vi "Update Intensity Plot.vi"(9 "Z":dbl[](array[numeric]), 10 "FEM Grid":T1, 11 "FEM plot in":refnum<vi>) -> (3 "FEM plot out":refnum<vi>)   [LabVIEW 2020, in "Heat Equation Solver.lvlib"]
uses:
  Heat Equation Solver.lvlib
  FEM Grid.ctl
  <vilib>/Analysis/baseanly.llb/Mean (DBL).vi
  <vilib>/picture/3D Picture Control/Object/Create Object (name).vi
  <vilib>/picture/3D Picture Control/NI_3D Picture Control.lvlib
  <vilib>/Analysis/NI_AALBase.lvlib
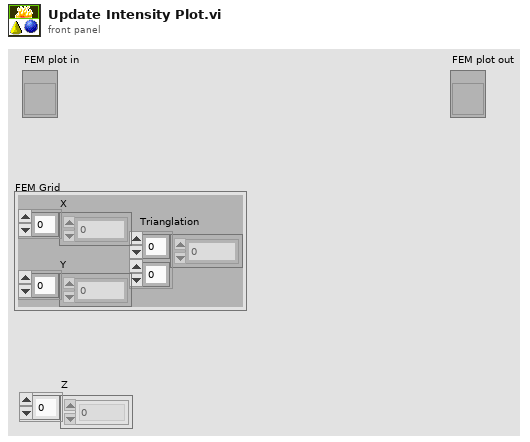
[diagram p1: front panel]
types:
  T1 = typedef "Heat Equation Solver.lvlib/FEM Grid.ctl" = cluster{"X":dbl[], "Y":dbl[], "Trianglation":i32[][]}
  T2 = enum16{"Inherit Value", "Points", "Wireframe", "Polygons"}
  T3 = enum16{"Overall", "Per Primitive", "Per Vertex", "Binding Off"}
  T4 = enum16{"Points", "Lines", "Line Strip", "Line Loop", "Triangles", "Triangle Strip", "Triangle Fan", "Quads", "Quad Strip", "Polygon"}
  T5 = cluster{"Numeric":dbl, "Numeric":dbl, "Numeric":dbl}
  T6 = typedef "LVRGBAColorTypeDef.ctl" = cluster{"Red":sgl, "Green":sgl, "Blue":sgl, "Alpha":sgl}
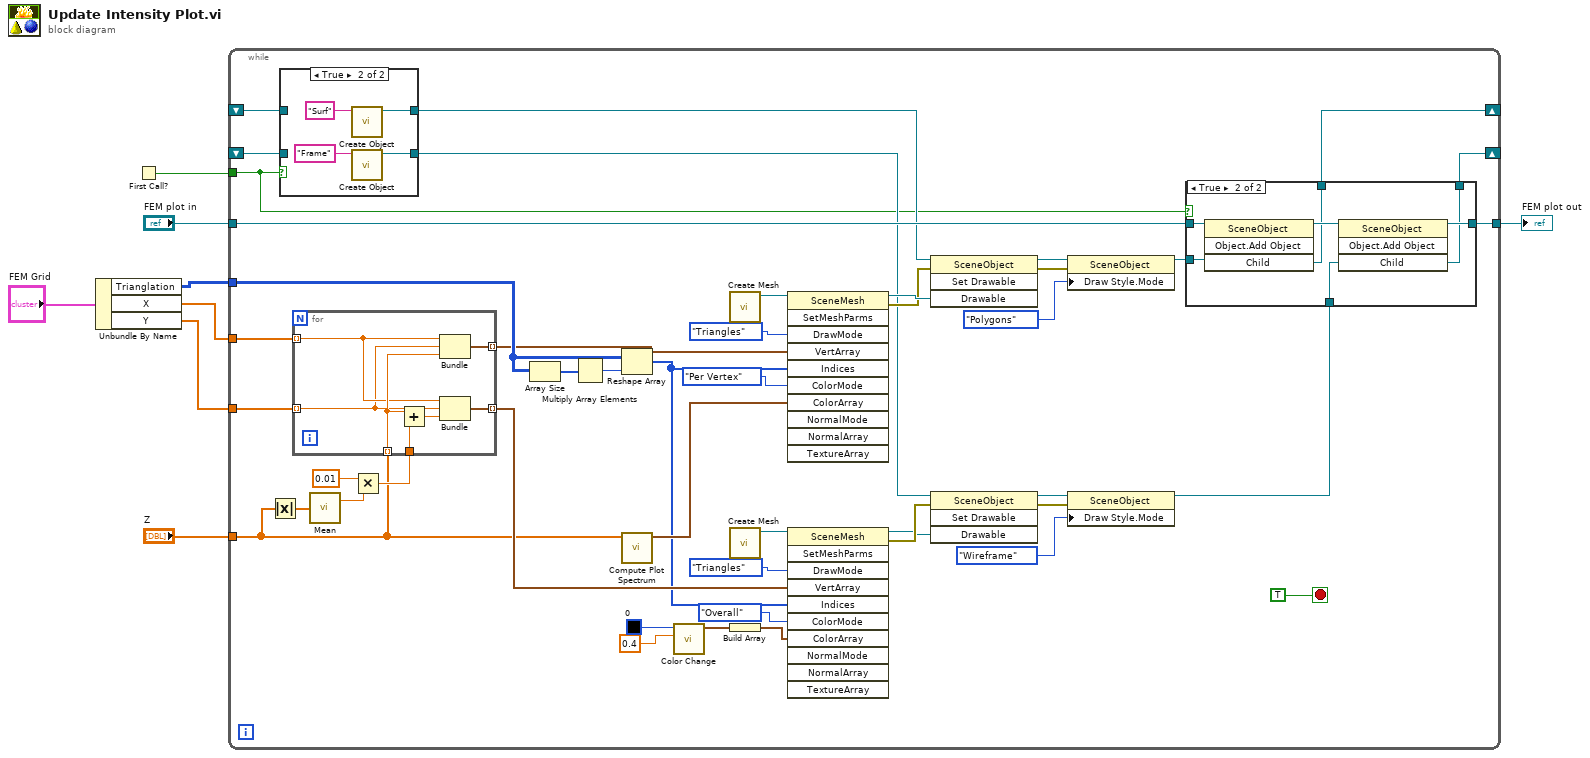
[diagram p0: block diagram]
diagram:
  n1 = Unbundle By Name("FEM Grid") -> ("Trianglation"=w3:i32[][], "X"=w2:dbl[], "Y"=w1:dbl[])
  n2 = First Call?() -> (First Call?: T/F=w5:bool)
  n3 = while {
    tunnel: w3 -> [w44]
    tunnel: "FEM plot in" -> [w25]
    tunnel: [w24] -> w7
    tunnel: "Z" -> [w19]
    tunnel: w2 -> [w18]
    tunnel: w1 -> [w17]
    tunnel: w5 -> [w11]
    shift-right: [w15] -> _
    shift-left: _ -> [w14]
    shift-right: [w12] -> _
    shift-left: _ -> [w10]
    stop <- TRUE stop-if-true
    n4 = Absolute Value(x=w19) -> (abs(x)=w20:dbl[])
    n5 = case shown="True" w11 {
      tunnel: [w66 w70] -> w16
      tunnel: w14 -> [w66 _]
      tunnel: [w65 w69] -> w13
      tunnel: w10 -> [w65 _]
      frame False {
      }
      frame True {
        n6 = call-poly <vilib>:"Create Object.vi"("Name"="Surf") -> ("Scene:New Object"=w70:refnum<vi>)  [unwired: 9 in, 1 out]
        n7 = call-poly <vilib>:"Create Object.vi"("Name"="Frame") -> ("Scene:New Object"=w69:refnum<vi>)  [unwired: 9 in, 1 out]
      }
    }
    n8 = call-poly <vilib>:"Mean.vi"("X"=w20) -> ("mean"=w23:dbl)  [unwired: 1 out]
    n9 = Multiply(x=0.01 ("y"), y=w23) -> (x*y=w21:dbl)
    n10 = for {
      tunnel: w19 -> [w76] mode=indexing
      tunnel: [w77] -> w34 mode=indexing
      tunnel: [w74] -> w33 mode=indexing
      tunnel: w21 -> [w73]
      tunnel: w18 -> [w72] mode=indexing
      tunnel: w17 -> [w71] mode=indexing
      n11 = Add(x=w76, y=w73) -> (x+y=w75:dbl)
      n12 = Bundle("Numeric"=w72, "Numeric"=w71, "Numeric"=w76) -> (w77:T5)  [unwired: 1 out]
      n13 = Bundle("Numeric"=w72, "Numeric"=w71, w75) -> (w74:cluster{"Numeric":dbl, "Numeric":dbl, dbl})  [unwired: 1 out]
    }
    n14 = Array Size(array=w44) -> (size(s)=w51:i32[])
    n15 = Multiply Array Elements(1:w51) -> (0:w50:i32)
    n16 = Reshape Array(w44, w50) -> (w32:i32[])
    n17 = call "Compute Plot Spectrum.vi"("U(x, y)"=w19) -> ("Color Array"=w45:T6[])  [unwired: 10 in]
    n18 = call <vilib>:"Color Change.vi"("Alpha"=0.4, "Color"=u32 0) -> ("RGBA"=w31:cluster{"R":sgl, "G":sgl, "B":sgl, "A":sgl})  [unwired: 9 in]
    n19 = call <vilib>:"Create Mesh.vi"() -> ("New Mesh Refnum"=w54:refnum<vi>)  [unwired: 1 in, 10 out]
    n20 = call <vilib>:"Create Mesh.vi"() -> ("New Mesh Refnum"=w35:refnum<vi>)  [unwired: 1 in, 10 out]
    n21 = Build Array(w31) -> (w30:cluster{"R":sgl, "G":sgl, "B":sgl, "A":sgl}[])
    n22 = invoke class="SceneMesh" method="SetMeshParms"(reference=w54, "DrawMode"=T4."Triangles" ("Draw Mode"), "VertArray"=w34, "Indices"=w32, "ColorMode"=T3."Per Vertex" ("Color Binding Mode"), "ColorArray"=w45) -> (reference out=w53:refnum<vi>, error out=w46:errorcluster)  [unwired: 5 in, 9 out]
    n23 = invoke class="SceneMesh" method="SetMeshParms"(reference=w35, "DrawMode"=T4."Triangles" ("Draw Mode"), "VertArray"=w33, "Indices"=w32, "ColorMode"=T3."Overall" ("Color Binding Mode"), "ColorArray"=w30) -> (reference out=w36:refnum<vi>, error out=w41:errorcluster)  [unwired: 5 in, 9 out]
    n24 = invoke class="SceneObject" method="Set Drawable"(reference=w16, error in=w46, "Drawable"=w53) -> (reference out=w52:refnum<vi>, error out=w47:errorcluster)  [unwired: 1 in, 2 out]
    n25 = invoke class="SceneObject" method="Set Drawable"(reference=w13, error in=w41, "Drawable"=w36) -> (reference out=w37:refnum<vi>, error out=w40:errorcluster)  [unwired: 1 in, 2 out]
    n26 = property class="SceneObject"(reference=w52, error in=w47, "Draw Style.Mode"=T2."Polygons" ("Draw Style:Mode")) -> (reference out=w27:refnum<vi>)  [unwired: 1 out]
    n27 = property class="SceneObject"(reference=w37, error in=w40, "Draw Style.Mode"=T2."Wireframe" ("Draw Style:Mode")) -> (reference out=w26:refnum<vi>)  [unwired: 1 out]
    n28 = case shown="True" w11 {
      tunnel: w27 -> [w57 w63]
      tunnel: w26 -> [w56 w62]
      tunnel: w25 -> [w55 w61]
      tunnel: [w55 w60] -> w24
      tunnel: [w57 w59] -> w15
      tunnel: [w56 w58] -> w12
      frame False {
      }
      frame True {
        n29 = invoke class="SceneObject" method="Object.Add Object"(reference=w61, "Child"=w63) -> (reference out=w64:refnum<vi>, "Child"=w59:refnum<vi>)  [unwired: 2 in, 2 out]
        n30 = invoke class="SceneObject" method="Object.Add Object"(reference=w64, "Child"=w62) -> (reference out=w60:refnum<vi>, "Child"=w58:refnum<vi>)  [unwired: 2 in, 2 out]
      }
    }
  }
  "FEM plot out" <- w7
